vi "Set Flow.vi"(8 "error in (no error)":errorcluster, 10 "State":bool, 11 "Main in":refnum<class "Main.lvclass">) -> (0 "error out":errorcluster, 3 "Main out":refnum<class "Main.lvclass">)   [LabVIEW 2018, in "Main.lvlib" / "Main.lvclass"]
uses:
  Main.lvclass
  Main.lvclass/Main.ctl
  Feeder Actor/Feeder Messages/Set Feeder Msg/Set Feeder Msg.lvclass/Set Feeder Msg.ctl
  <vilib>/ActorFramework/Message Enqueuer/Message Enqueuer.lvclass/Message Enqueuer.ctl
  <vilib>/ActorFramework/Message Enqueuer/Enqueue.vi
  Feeder Actor/Feeder Messages/Set Feeder Msg/Set Feeder Msg.lvclass
  C:/Program Files/National Instruments/LabVIEW 2018/vi.lib/ActorFramework/Message/Message.lvclass
  <vilib>/ActorFramework/Message Priority Queue/Priority Enqueue.vi
  MFC Actor/MFC Messages/Set Print Msg/Set Print Msg.lvclass
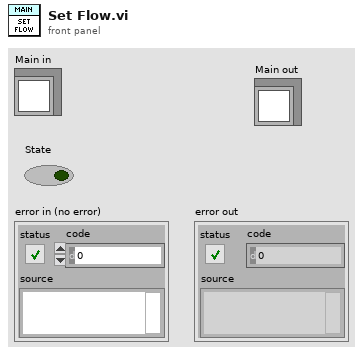
[diagram p1: front panel]
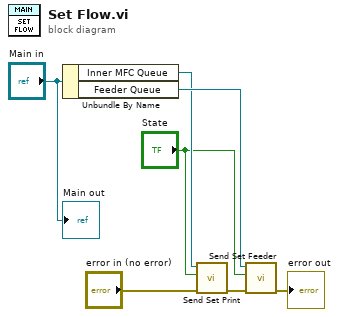
[diagram p0: block diagram]
diagram:
  n1 = Unbundle By Name("Main in") -> ("Inner MFC Queue"=w4:refnum<class "Message Enqueuer.lvclass">, "Feeder Queue"=w6:refnum<class "Message Enqueuer.lvclass">)
  n2 = call "Send Set Print.vi"("error in (no error)"="error in (no error)", "On?"="State", "Message Enqueuer in"=w4) -> ("error out"=w2:errorcluster)  [unwired: 7 in, 1 out]
  n3 = call "Send Set Feeder.vi"("error in (no error)"=w2, "State"="State", "Message Enqueuer in"=w6) -> ("error out"=→"error out":errorcluster)  [unwired: 7 in, 1 out]
  "Main out" <- "Main in"
